vi "HoloPy_sum_XY_planes_from_volume.vi"(8 "error in (no error)":errorcluster, 11 "Refnum in":refnum<k35>) -> (0 "error out":errorcluster, 2 "XY Plane":sgl[][](array[numeric]), 3 "Refnum out":refnum<k35>)   [LabVIEW 2023, in "holoPyTracks.lvlib"]
uses:
  holoPyTracks.lvlib
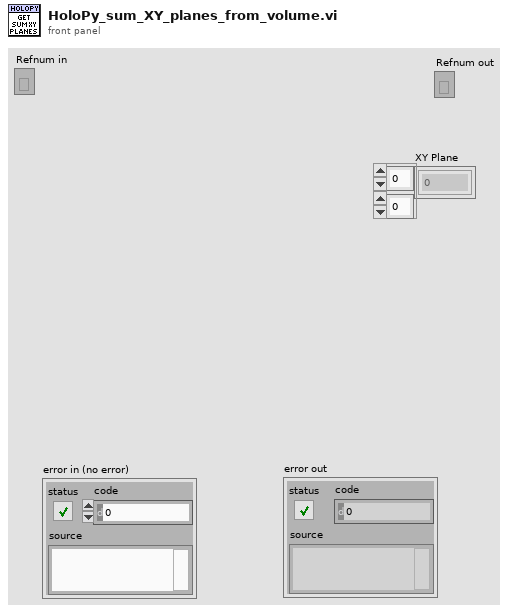
[diagram p1: front panel]
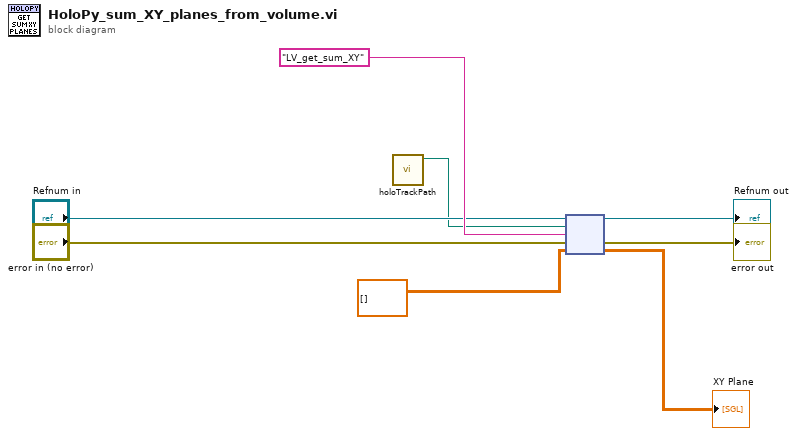
[diagram p0: block diagram]
diagram:
  n1 = call "holoTrackPath.vi"() -> ("appended path"=w1:path)  [unwired: 11 in]
  n2 = node("Refnum in", w1, "LV_get_sum_XY" ("function name"), "error in (no error)", sgl[][] []) -> (→"Refnum out":refnum<k35>, →"error out":errorcluster, →"XY Plane":sgl[][])  [unwired: 2 out]
